vi "Log.vi"(0 "Iterationer":dbl[](array[numeric]), 2 "Rumtemperatur":dbl[](array[numeric]), 4 "Slush Ice":dbl[](array[numeric]), 6 "Brine":dbl[](array[numeric]), 7 "output cluster":T1, 11 "Motor":dbl[](array[numeric]), 14 "Efter ForD":dbl[](array[numeric]), 15 "Kond luft":dbl[](array[numeric]), 18 "Komp":dbl[](array[numeric]), 19 "Efter EPV":dbl[](array[numeric]), 20 "Efter Komp":dbl[](array[numeric]), 22 "Efter Kond":dbl[](array[numeric]), 24 "Tryk hoej":dbl[](array[numeric]), 26 "Tryk lav":dbl[](array[numeric])) -> ()   [LabVIEW 2022 SP3]
uses:
  TypeDefs/CoolPropArrays.ctl
  TypeDefs/CoolPropArrayData.ctl
  <vilib>/Utility/file.llb/Write Delimited Spreadsheet (string).vi
panel:
  in  "Efter Kond":dbl[](array[numeric])
  out "transposed array":string[][](array[string])
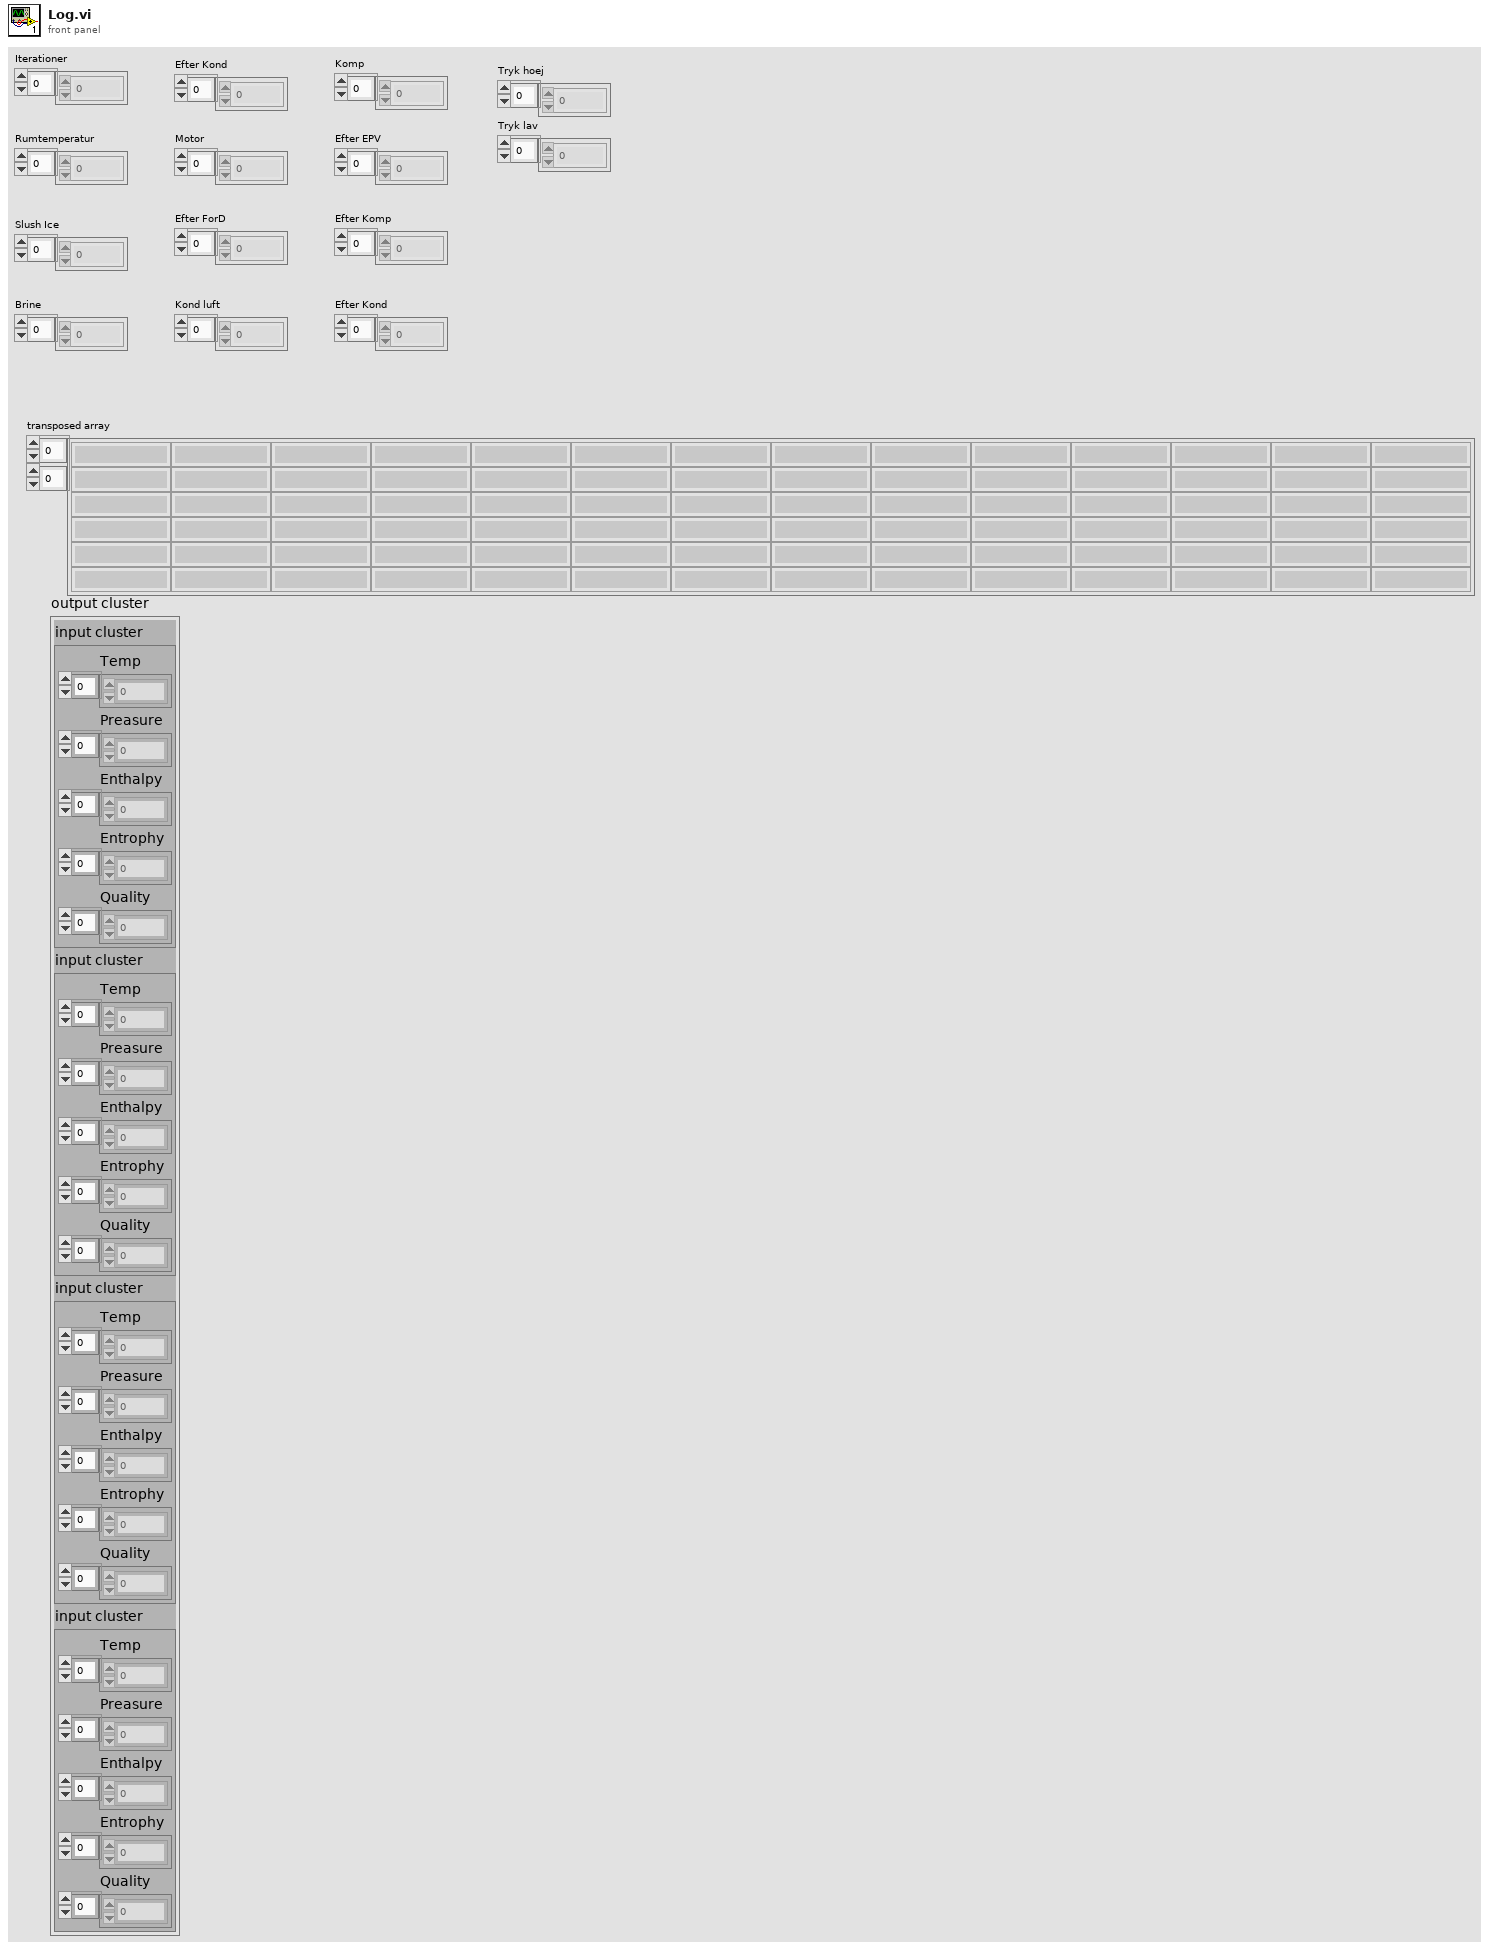
[diagram p1: front panel]
types:
  T1 = typedef "CoolPropArrays.ctl" = cluster{"input cluster":T2, "input cluster":T2, "input cluster":T2, "input cluster":T2}
  T2 = typedef "CoolPropArrayData.ctl" = cluster{"Temp":dbl[], "Preasure":dbl[], "Enthalpy":dbl[], "Entrophy":dbl[], "Quality":dbl[]}
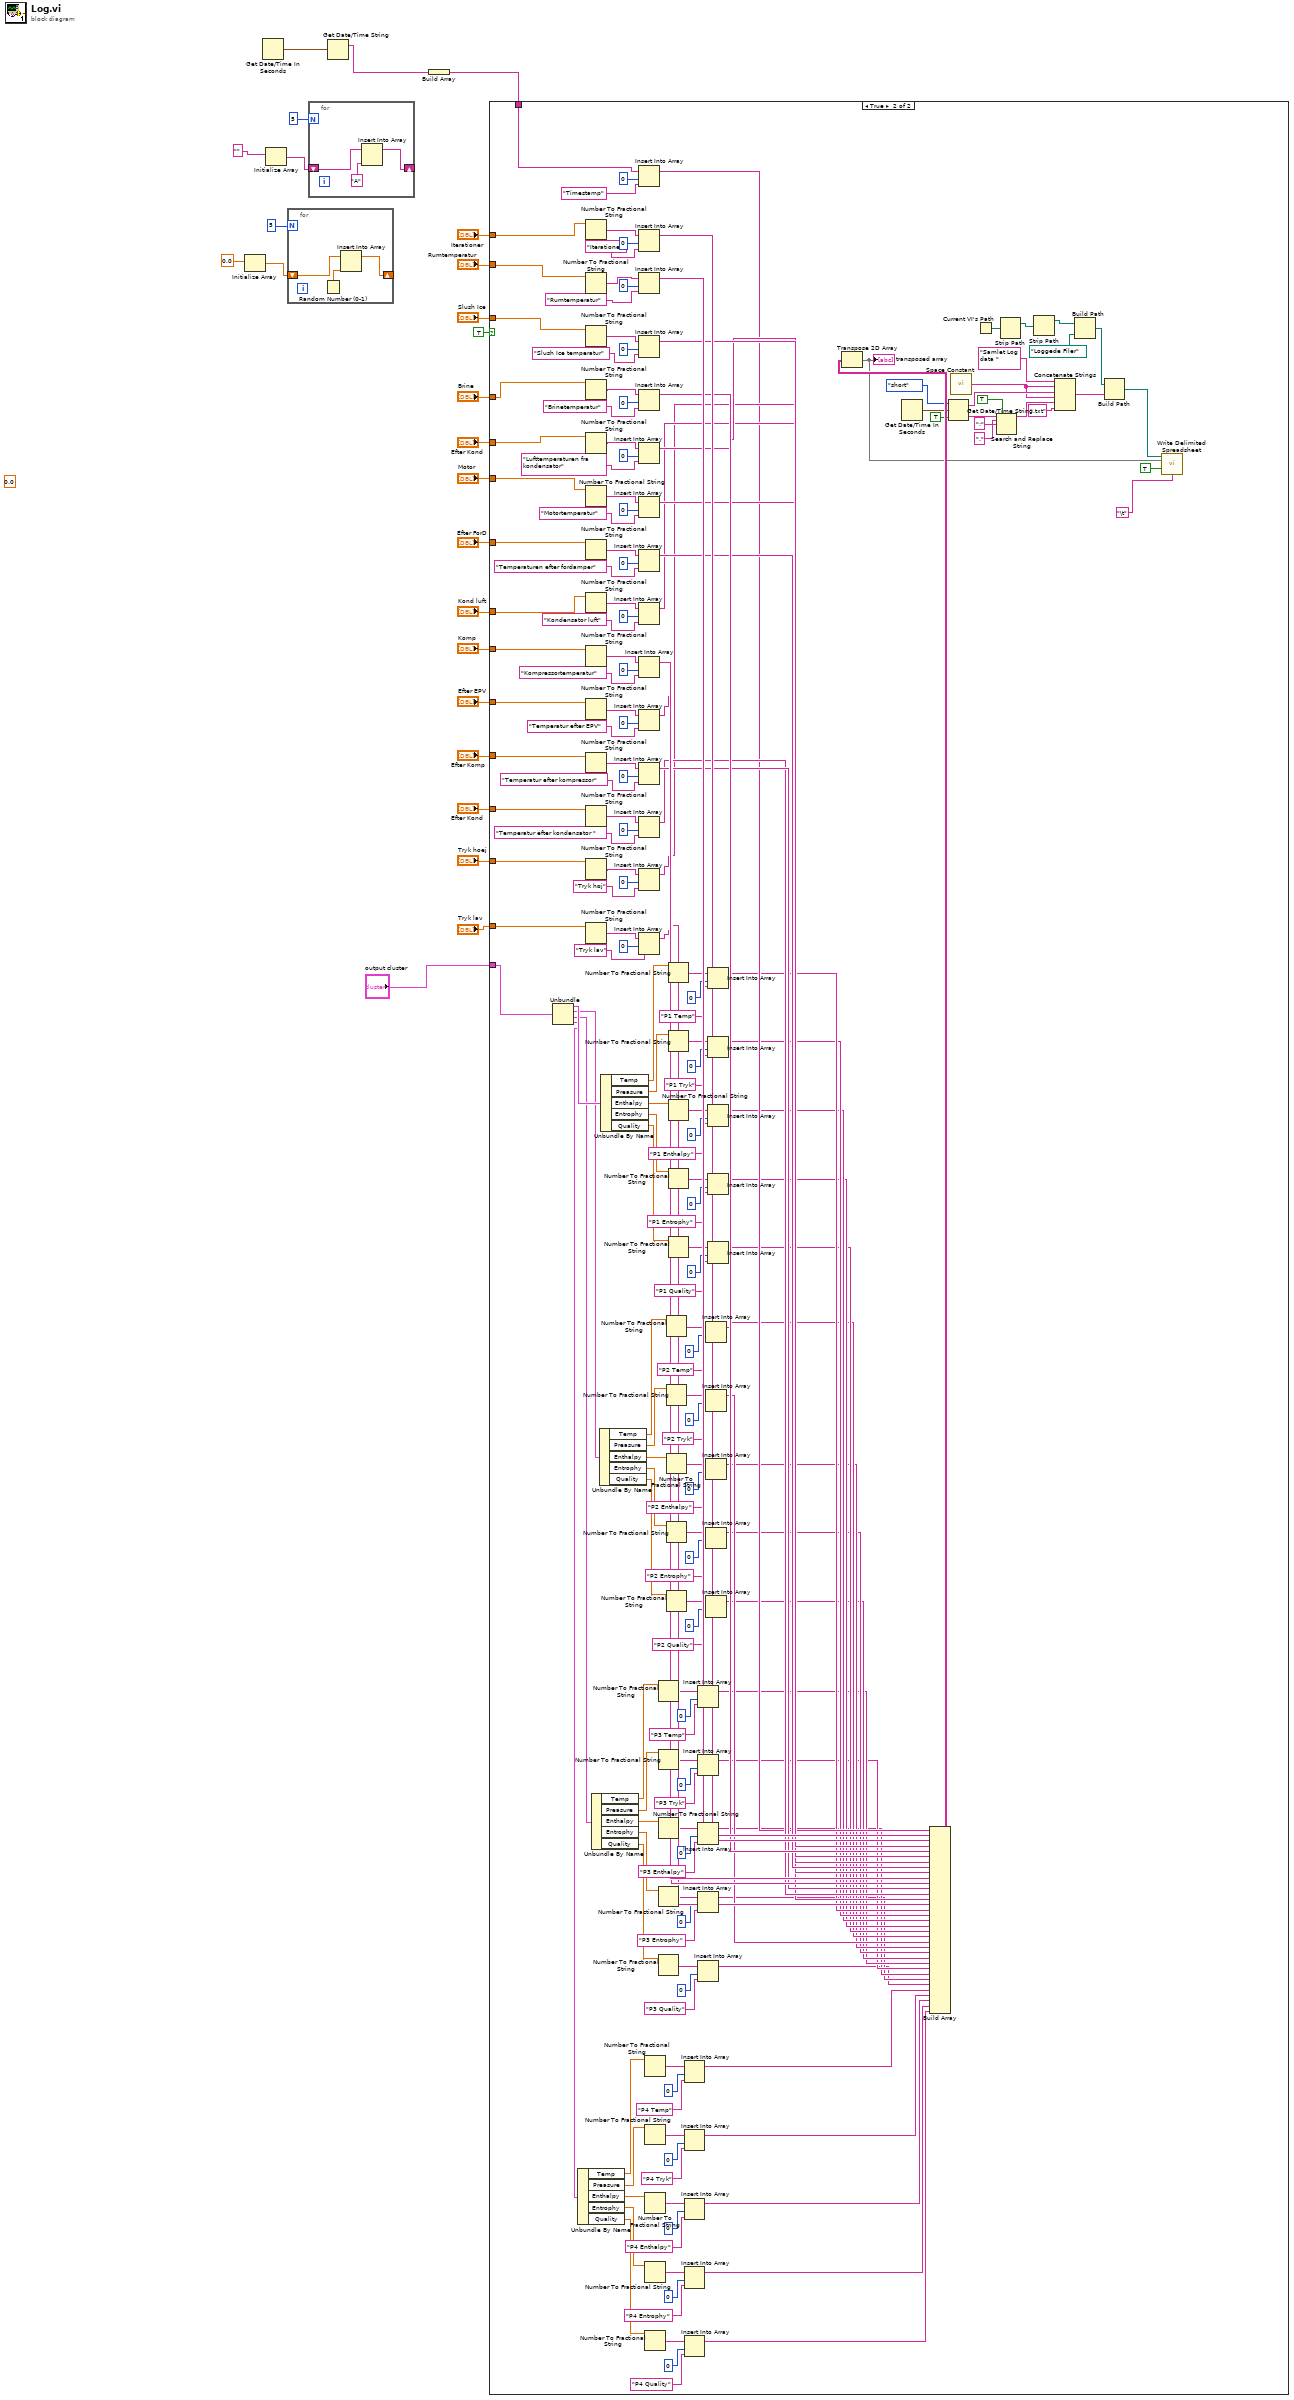
[diagram p0: block diagram]
diagram:
  (unwired) 0.0 ("element")
  n1 = Initialize Array(0.0 ("element")) -> (w25:dbl[])  [unwired: 1 in]
  n2 = Get Date/Time In Seconds() -> (seconds since 1Jan1904=w4:timestamp)
  n3 = Initialize Array("") -> (w19:string[])  [unwired: 1 in]
  n4 = for {
    N: 5 -> [_]
    shift-right: [w27] -> _
    shift-left: w25 -> [w28]
    n5 = Random Number (0-1)() -> (number: 0 to 1=w26:dbl)
    n6 = Insert Into Array(array=w28, new element=w26) -> (w27:dbl[])  [unwired: 1 in]
  }
  n7 = for {
    N: 5 -> [_]
    shift-right: [w31] -> _
    shift-left: w19 -> [w29]
    n8 = Insert Into Array(array=w29, new element="A") -> (w31:string[])  [unwired: 1 in]
  }
  n9 = Get Date/Time String(seconds (now)=w4) -> (date string=w3:string)  [unwired: 2 in, 1 out]
  n10 = Build Array(w3) -> (w2:string[])
  n11 = case shown="True" TRUE {
    tunnel: "Rumtemperatur" -> [_ w232]
    tunnel: "Iterationer" -> [_ w233]
    tunnel: "Slush Ice" -> [_ w231]
    tunnel: "Brine" -> [_ w230]
    tunnel: "Motor" -> [_ w229]
    tunnel: "Efter ForD" -> [_ w228]
    tunnel: "Kond luft" -> [_ w227]
    tunnel: "Komp" -> [_ w226]
    tunnel: "Efter EPV" -> [_ w225]
    tunnel: "Efter Komp" -> [_ w224]
    tunnel: "Efter Kond" -> [_ w223]
    tunnel: "Efter Kond" -> [_ w222]
    tunnel: "Tryk lav" -> [_ w139]
    tunnel: "Tryk hoej" -> [_ w138]
    tunnel: w2 -> [_ w137]
    tunnel: "output cluster" -> [_ w136]
    frame False {
    }
    frame True {
      n12 = Unbundle(w136) -> ("input cluster"=w135:T2, "input cluster"=w94:T2, "input cluster"=w73:T2, "input cluster"=w52:T2)
      n13 = Unbundle By Name(w52) -> ("Temp"=w69:dbl[], "Preasure"=w56:dbl[], "Enthalpy"=w55:dbl[], "Entrophy"=w54:dbl[], "Quality"=w53:dbl[])
      n14 = Number To Fractional String(number=w233) -> (F-format string=w220:string[])  [unwired: 3 in]
      n15 = Number To Fractional String(number=w232) -> (F-format string=w216:string[])  [unwired: 3 in]
      n16 = Number To Fractional String(number=w231) -> (F-format string=w204:string[])  [unwired: 3 in]
      n17 = Number To Fractional String(number=w230) -> (F-format string=w202:string[])  [unwired: 3 in]
      n18 = Number To Fractional String(number=w222) -> (F-format string=w200:string[])  [unwired: 3 in]
      n19 = Number To Fractional String(number=w229) -> (F-format string=w198:string[])  [unwired: 3 in]
      n20 = Number To Fractional String(number=w228) -> (F-format string=w196:string[])  [unwired: 3 in]
      n21 = Number To Fractional String(number=w227) -> (F-format string=w193:string[])  [unwired: 3 in]
      n22 = Number To Fractional String(number=w226) -> (F-format string=w189:string[])  [unwired: 3 in]
      n23 = Number To Fractional String(number=w225) -> (F-format string=w190:string[])  [unwired: 3 in]
      n24 = Number To Fractional String(number=w224) -> (F-format string=w187:string[])  [unwired: 3 in]
      n25 = Number To Fractional String(number=w223) -> (F-format string=w185:string[])  [unwired: 3 in]
      n26 = Number To Fractional String(number=w138) -> (F-format string=w184:string[])  [unwired: 3 in]
      n27 = Number To Fractional String(number=w139) -> (F-format string=w181:string[])  [unwired: 3 in]
      n28 = Unbundle By Name(w73) -> ("Temp"=w90:dbl[], "Preasure"=w77:dbl[], "Enthalpy"=w76:dbl[], "Entrophy"=w75:dbl[], "Quality"=w74:dbl[])
      n29 = Unbundle By Name(w94) -> ("Temp"=w111:dbl[], "Preasure"=w98:dbl[], "Enthalpy"=w97:dbl[], "Entrophy"=w96:dbl[], "Quality"=w95:dbl[])
      n30 = Unbundle By Name(w135) -> ("Temp"=w131:dbl[], "Preasure"=w118:dbl[], "Enthalpy"=w117:dbl[], "Entrophy"=w116:dbl[], "Quality"=w115:dbl[])
      n31 = Insert Into Array(array=w137, index=0 ("index (row)"), new element="Timestamp") -> (w144:string[])
      n32 = Insert Into Array(array=w220, index=0 ("index (row)"), new element="Iterationer") -> (w179:string[])
      n33 = Insert Into Array(array=w216, index=0 ("index (row)"), new element="Rumtemperatur") -> (w178:string[])
      n34 = Insert Into Array(array=w204, index=0 ("index (row)"), new element="Slush Ice temperatur") -> (w177:string[])
      n35 = Insert Into Array(array=w202, index=0 ("index (row)"), new element="Brinetemperatur" ("element")) -> (w176:string[])
      n36 = Insert Into Array(array=w200, index=0 ("index (row)"), new element="Lufttemperaturen fra kondensator" ("element")) -> (w175:string[])
      n37 = Insert Into Array(array=w198, index=0 ("index (row)"), new element="Motortemperatur" ("element")) -> (w174:string[])
      n38 = Insert Into Array(array=w196, index=0 ("index (row)"), new element="Temperaturen efter fordamper" ("element")) -> (w173:string[])
      n39 = Insert Into Array(array=w193, index=0 ("index (row)"), new element="Kondensator luft" ("element")) -> (w172:string[])
      n40 = Insert Into Array(array=w189, index=0 ("index (row)"), new element="Kompressortemperatur" ("element")) -> (w171:string[])
      n41 = Insert Into Array(array=w190, index=0 ("index (row)"), new element="Temperatur efter EPV" ("element")) -> (w170:string[])
      n42 = Insert Into Array(array=w187, index=0 ("index (row)"), new element="Temperatur efter kompressor" ("element")) -> (w169:string[])
      n43 = Insert Into Array(array=w185, index=0 ("index (row)"), new element="Temperatur efter kondensator " ("element")) -> (w168:string[])
      n44 = Insert Into Array(array=w184, index=0 ("index (row)"), new element="Tryk høj" ("element")) -> (w167:string[])
      n45 = Insert Into Array(array=w181, index=0 ("index (row)"), new element="Tryk lav" ("element")) -> (w166:string[])
      n46 = Number To Fractional String(number=w69) -> (F-format string=w71:string[])  [unwired: 3 in]
      n47 = Number To Fractional String(number=w56) -> (F-format string=w67:string[])  [unwired: 3 in]
      n48 = Number To Fractional String(number=w55) -> (F-format string=w64:string[])  [unwired: 3 in]
      n49 = Number To Fractional String(number=w54) -> (F-format string=w61:string[])  [unwired: 3 in]
      n50 = Number To Fractional String(number=w53) -> (F-format string=w58:string[])  [unwired: 3 in]
      n51 = Number To Fractional String(number=w90) -> (F-format string=w92:string[])  [unwired: 3 in]
      n52 = Number To Fractional String(number=w77) -> (F-format string=w88:string[])  [unwired: 3 in]
      n53 = Number To Fractional String(number=w76) -> (F-format string=w85:string[])  [unwired: 3 in]
      n54 = Number To Fractional String(number=w75) -> (F-format string=w82:string[])  [unwired: 3 in]
      n55 = Number To Fractional String(number=w74) -> (F-format string=w79:string[])  [unwired: 3 in]
      n56 = Number To Fractional String(number=w111) -> (F-format string=w113:string[])  [unwired: 3 in]
      n57 = Number To Fractional String(number=w98) -> (F-format string=w109:string[])  [unwired: 3 in]
      n58 = Number To Fractional String(number=w97) -> (F-format string=w106:string[])  [unwired: 3 in]
      n59 = Number To Fractional String(number=w96) -> (F-format string=w103:string[])  [unwired: 3 in]
      n60 = Number To Fractional String(number=w95) -> (F-format string=w100:string[])  [unwired: 3 in]
      n61 = Number To Fractional String(number=w131) -> (F-format string=w133:string[])  [unwired: 3 in]
      n62 = Number To Fractional String(number=w118) -> (F-format string=w129:string[])  [unwired: 3 in]
      n63 = Number To Fractional String(number=w117) -> (F-format string=w126:string[])  [unwired: 3 in]
      n64 = Number To Fractional String(number=w116) -> (F-format string=w123:string[])  [unwired: 3 in]
      n65 = Number To Fractional String(number=w115) -> (F-format string=w120:string[])  [unwired: 3 in]
      n66 = Insert Into Array(array=w71, index=0 ("index (row)"), new element="P4 Temp" ("element")) -> (w36:string[])
      n67 = Insert Into Array(array=w67, index=0 ("index (row)"), new element="P4 Tryk" ("element")) -> (w35:string[])
      n68 = Insert Into Array(array=w64, index=0 ("index (row)"), new element="P4 Enthalpy" ("element")) -> (w34:string[])
      n69 = Insert Into Array(array=w61, index=0 ("index (row)"), new element="P4 Entrophy" ("element")) -> (w33:string[])
      n70 = Insert Into Array(array=w58, index=0 ("index (row)"), new element="P4 Quality" ("element")) -> (w32:string[])
      n71 = Insert Into Array(array=w92, index=0 ("index (row)"), new element="P3 Temp" ("element")) -> (w41:string[])
      n72 = Insert Into Array(array=w88, index=0 ("index (row)"), new element="P3 Tryk" ("element")) -> (w40:string[])
      n73 = Insert Into Array(array=w85, index=0 ("index (row)"), new element="P3 Enthalpy" ("element")) -> (w39:string[])
      n74 = Insert Into Array(array=w82, index=0 ("index (row)"), new element="P3 Entrophy" ("element")) -> (w38:string[])
      n75 = Insert Into Array(array=w79, index=0 ("index (row)"), new element="P3 Quality" ("element")) -> (w37:string[])
      n76 = Insert Into Array(array=w113, index=0 ("index (row)"), new element="P2 Temp" ("element")) -> (w46:string[])
      n77 = Insert Into Array(array=w109, index=0 ("index (row)"), new element="P2 Tryk" ("element")) -> (w45:string[])
      n78 = Insert Into Array(array=w106, index=0 ("index (row)"), new element="P2 Enthalpy" ("element")) -> (w44:string[])
      n79 = Insert Into Array(array=w103, index=0 ("index (row)"), new element="P2 Entrophy" ("element")) -> (w43:string[])
      n80 = Insert Into Array(array=w100, index=0 ("index (row)"), new element="P2 Quality" ("element")) -> (w42:string[])
      n81 = Insert Into Array(array=w133, index=0 ("index (row)"), new element="P1 Temp" ("element")) -> (w51:string[])
      n82 = Insert Into Array(array=w129, index=0 ("index (row)"), new element="P1 Tryk" ("element")) -> (w50:string[])
      n83 = Insert Into Array(array=w126, index=0 ("index (row)"), new element="P1 Enthalpy" ("element")) -> (w49:string[])
      n84 = Insert Into Array(array=w123, index=0 ("index (row)"), new element="P1 Entrophy" ("element")) -> (w48:string[])
      n85 = Insert Into Array(array=w120, index=0 ("index (row)"), new element="P1 Quality" ("element")) -> (w47:string[])
      n86 = Get Date/Time In Seconds() -> (seconds since 1Jan1904=w154:timestamp)
      n87 = Build Array(w144, w179, w178, w177, w176, w175, w174, w173, w172, w171, w170, w169, w168, w167, w166, w51, w50, w49, w48, w47, w46, w45, w44, w43, w42, w41, w40, w39, w38, w37, w36, w35, w34, w33, w32) -> (w165:string[][])
      n88 = Transpose 2D Array(2D array=w165) -> (transposed array=w164:string[][])
      "transposed array" <- w164
      n89 = Get Date/Time String(date format (0)=enum16{"short", "long", "abbreviated"}."short", seconds (now)=w154, want seconds? (F)=TRUE) -> (date string=w151:string, time string=w157:string)
      n90 = call <vilib>:"Space Constant.vi"() -> ("String"=w150:string)
      n91 = Current VI's Path() -> (path=w163:path)
      n92 = Search and Replace String(replace all?=TRUE ("replace all? (F)"), input string=w157, search string=":", replace string="." ("replace string (\"\")")) -> (result string=w149:string)  [unwired: 4 in, 3 out]
      n93 = Strip Path(path=w163) -> (stripped path=w143:path)  [unwired: 1 out]
      n94 = Strip Path(path=w143) -> (stripped path=w142:path)  [unwired: 1 out]
      n95 = Concatenate Strings("Samlet Log data " ("string"), w150, w151, w150, w149, ".txt" ("string")) -> (w161:string)
      n96 = Build Path(base path=w142, name or relative path=path "Loggede Filer") -> (appended path=w152:path)
      n97 = Build Path(base path=w152, name or relative path=w161) -> (appended path=w147:path)
      n98 = call-poly <vilib>:"Write Delimited Spreadsheet.vi"("file path (dialog if empty)"=w147, "2D data"=w164, "append to file? (new file:F)"=TRUE, "delimiter (\\t)"="\t") -> ()  [unwired: 10 in, 2 out]
    }
  }
